vi "关键参数存表.vi"(7 "table":string="3090仪器参数", 8 "error in (no error)":errorcluster, 9 "仪器参数":T2, 10 "datatime":timestamp, 11 "仪器名称":string) -> (0 "error out":errorcluster)   [LabVIEW 2016, in "斯坦道CODcr.lvlib"]
panel:
  out "data in":T1
  in  "database":string="database3.mdb"
  out "columns":string[](array[string])
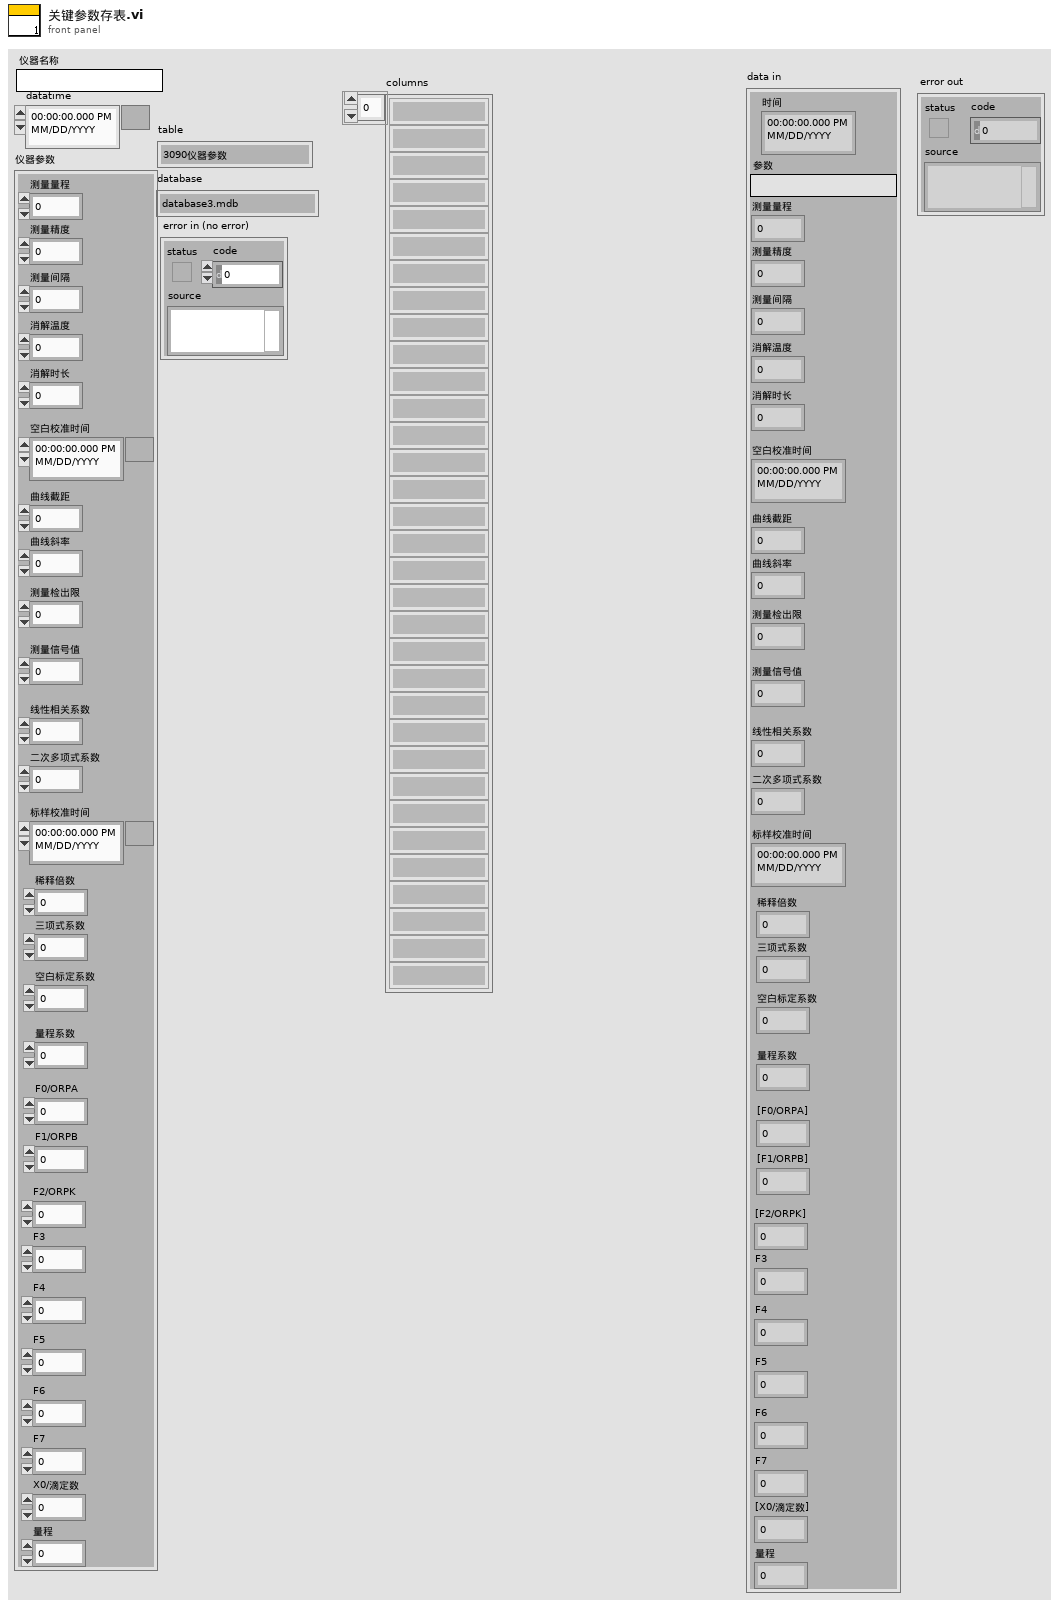
[diagram p1: front panel]
types:
  T1 = cluster{"时间":timestamp, "参数":string, "测量量程":dbl, "测量精度":dbl, "测量间隔":dbl, "消解温度":dbl, "消解时长":dbl, "空白校准时间":timestamp, "曲线截距":dbl, "曲线斜率":dbl, "测量检出限":dbl, "测量信号值":dbl, "线性相关系数":dbl, "二次多项式系数":dbl, "标样校准时间":timestamp, "稀释倍数":dbl, "三项式系数":dbl, "空白标定系数":dbl, "量程系数":dbl, "[F0/ORPA]":dbl, "[F1/ORPB]":dbl, "[F2/ORPK]":dbl, "F3":dbl, "F4":dbl, "F5":dbl, "F6":dbl, "F7":dbl, "[X0/滴定数]":dbl, "量程":dbl}
  T2 = cluster{"测量量程":dbl, "测量精度":dbl, "测量间隔":dbl, "消解温度":dbl, "消解时长":dbl, "空白校准时间":timestamp, "曲线截距":dbl, "曲线斜率":dbl, "测量检出限":dbl, "测量信号值":dbl, "线性相关系数":dbl, "二次多项式系数":dbl, "标样校准时间":timestamp, "稀释倍数":dbl, "三项式系数":dbl, "空白标定系数":dbl, "量程系数":dbl, "F0/ORPA":dbl, "F1/ORPB":dbl, "F2/ORPK":dbl, "F3":dbl, "F4":dbl, "F5":dbl, "F6":dbl, "F7":dbl, "X0/滴定数":dbl, "量程":dbl}
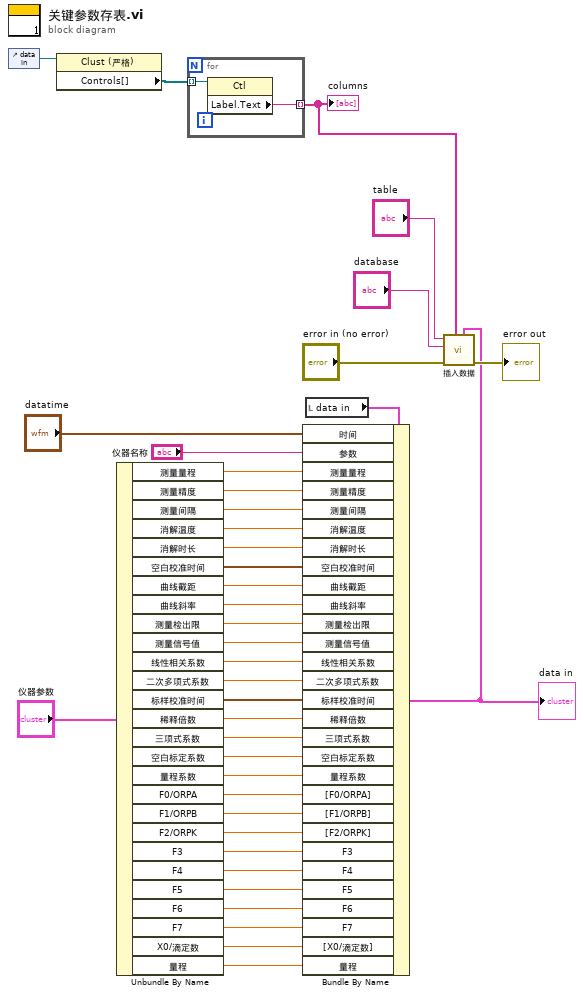
[diagram p0: block diagram]
diagram:
  n1 = control-ref of="data in"() -> (w17:refnum<vi>)
  n2 = property class="Clust (严格)"(reference=w17) -> ("Controls[]"=w16:refnum<vi>[])  [unwired: 1 in, 2 out]
  n3 = Unbundle By Name("仪器参数") -> ("测量量程"=w39:dbl, "测量精度"=w38:dbl, "测量间隔"=w37:dbl, "消解温度"=w36:dbl, "消解时长"=w35:dbl, "空白校准时间"=w34:timestamp, "曲线截距"=w33:dbl, "曲线斜率"=w32:dbl, "测量检出限"=w31:dbl, "测量信号值"=w30:dbl, "线性相关系数"=w29:dbl, "二次多项式系数"=w28:dbl, "标样校准时间"=w27:timestamp, "稀释倍数"=w14:dbl, "三项式系数"=w13:dbl, "空白标定系数"=w12:dbl, "量程系数"=w11:dbl, "F0/ORPA"=w10:dbl, "F1/ORPB"=w9:dbl, "F2/ORPK"=w8:dbl, "F3"=w7:dbl, "F4"=w6:dbl, "F5"=w5:dbl, "F6"=w4:dbl, "F7"=w3:dbl, "X0/滴定数"=w2:dbl, "量程"=w1:dbl)
  n4 = for {
    tunnel: w16 -> [w41] mode=indexing
    tunnel: [w40] -> w18 mode=indexing
    n5 = property class="Ctl"(reference=w41) -> ("Label.Text"=w40:string)  [unwired: 1 in, 2 out]
  }
  "columns" <- w18
  n6 = local read "data in"() -> (w25:T1)
  n7 = Bundle By Name(cluster=w25, "时间"="datatime", "参数"="仪器名称", "测量量程"=w39, "测量精度"=w38, "测量间隔"=w37, "消解温度"=w36, "消解时长"=w35, "空白校准时间"=w34, "曲线截距"=w33, "曲线斜率"=w32, "测量检出限"=w31, "测量信号值"=w30, "线性相关系数"=w29, "二次多项式系数"=w28, "标样校准时间"=w27, "稀释倍数"=w14, "三项式系数"=w13, "空白标定系数"=w12, "量程系数"=w11, "[F0/ORPA]"=w10, "[F1/ORPB]"=w9, "[F2/ORPK]"=w8, "F3"=w7, "F4"=w6, "F5"=w5, "F6"=w4, "F7"=w3, "[X0/滴定数]"=w2, "量程"=w1) -> (w19:T1)
  "data in" <- w19
  n8 = call "插入数据.vi"("data"=w19, "columns"=w18, "error in (no error)"="error in (no error)", "database"="database", "table"="table") -> ("error out"=→"error out":errorcluster)  [unwired: 6 in]
